vi "SAWparms after fit.vi"(8 "x array":dbl[](array[numeric]), 9 "best fit y":dbl[](array[numeric]), 11 "best fit parms":dbl[](array[numeric])) -> (0 "Q factor":dbl, 1 "Bandwidth":dbl, 2 "S11 dip":dbl, 3 "fc from fit":dbl)   [LabVIEW 2020]
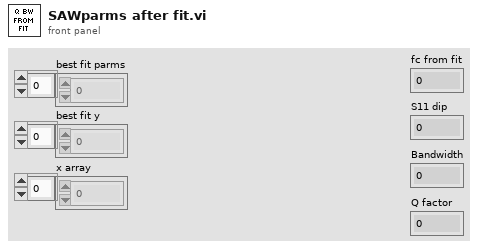
[diagram p1: front panel]
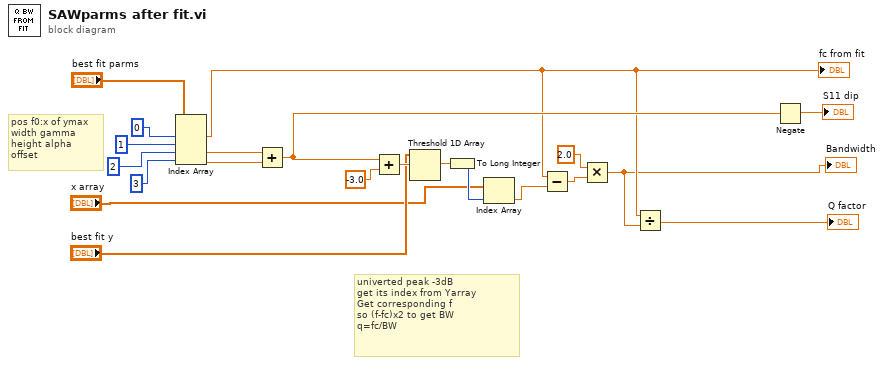
[diagram p0: block diagram]
diagram:
  # "pos f0:x of ymax\nwidth gamma\nheight alpha\noffset"
  # "univerted peak -3dB\nget its index from Yarray\nGet corresponding f\nso (f-fc)x2 to get BW\nq=fc/BW"
  n1 = Index Array(array="best fit parms", index #1=0 ("index"), index #2=1 ("index"), index #3=2 ("index"), index #4=3 ("index")) -> (element #1=w3:dbl, element #3=w17:dbl, element #4=w16:dbl)  [unwired: 1 out]
  "fc from fit" <- w3
  n2 = Add(x=w17, y=w16) -> (x+y=w14:dbl)
  n3 = Add(x=w14, y=-3.0) -> (x+y=w15:dbl)
  n4 = Threshold 1D Array(2:w15, 3:"best fit y") -> (0:w11:dbl)  [unwired: 1 in]
  n5 = To Long Integer(number=w11) -> (32bit integer=w12:i32)
  n6 = Index Array(array="x array", index=w12) -> (element=w6:dbl)
  n7 = Subtract(x=w3, y=w6) -> (x-y=w5:dbl)
  n8 = Multiply(x=2.0, y=w5) -> (x*y=w2:dbl)
  "Bandwidth" <- w2
  n9 = Divide(x=w3, y=w2) -> (x/y=→"Q factor":dbl)
  n10 = Negate(x=w14) -> (-x=→"S11 dip":dbl)
